vi "Initialize.vi"(8 "error in (no error)":errorcluster caption="错误输入（无错误）", 10 "Reset? (T: Reset)":bool=TRUE, 11 "Keithley 2000 输入":refnum<class "Keithley 2000.lvclass">) -> (0 "error out":errorcluster caption="错误输出", 3 "Keithley 2000 输出":refnum<class "Keithley 2000.lvclass">)   [LabVIEW 2020, in "DMM.lvlib" / "Keithley 2000.lvclass"]
uses:
  Keithley 2000.lvclass
  D:/LVProject/Class/LVDevClass/DMM/root/DMM.lvclass
  Keithley 2000.lvclass/Keithley 2000.ctl
  <instrlib>/Keithley 2000/Keithley 2000.lvlib
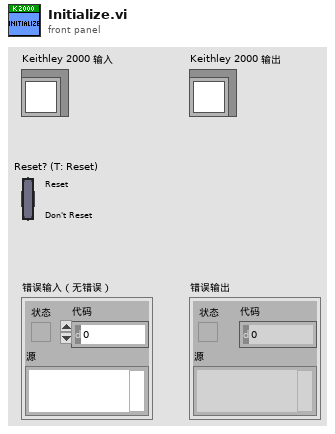
[diagram p1: front panel]
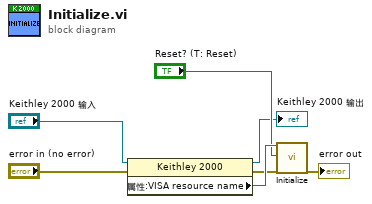
[diagram p0: block diagram]
diagram:
  n1 = property class="Keithley 2000"(reference="Keithley 2000 输入", error in="error in (no error)") -> (reference out=→"Keithley 2000 输出":refnum<class "Keithley 2000.lvclass">, error out=w3:errorcluster, "属性:VISA resource name"=w5:refnum<visa-resource-name>)
  n2 = call <instrlib>:"Initialize.vi"("VISA resource name"=w5, "Reset? (T: Reset)"="Reset? (T: Reset)", "error in (no error)"=w3) -> ("error out"=→"error out":errorcluster)  [unwired: 15 in, 1 out]
